vi "GetAllPropertyName.vi"(11 "JSON":string) -> (3 "output array":string[](array[string]))   [LabVIEW 2017]
uses:
  <vilib>/JDP Science/JSONtext/JSONtext.lvlib
  69925c48-c7bb-4434-a24c-5319c87c29c6.vi
  955f1e7d-53c6-494f-b1ae-88a05e9839de.vi
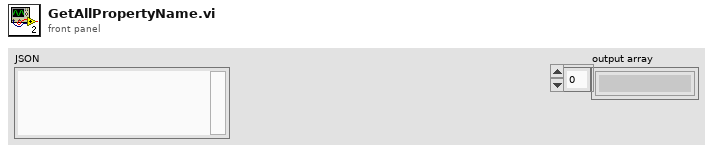
[diagram p1: front panel]
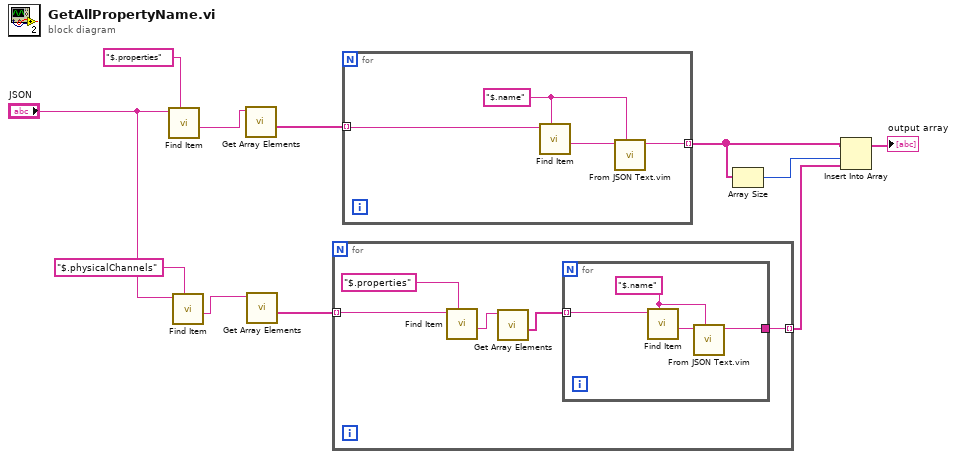
[diagram p0: block diagram]
diagram:
  n1 = call <vilib>:"Find Item.vi"("$Path or Item Name"="$.properties", "JSON"="JSON") -> ("<JSON>"=w10:string)  [unwired: 6 in, 3 out]
  n2 = call <vilib>:"Find Item.vi"("$Path or Item Name"="$.physicalChannels", "JSON"="JSON") -> ("<JSON>"=w6:string)  [unwired: 6 in, 3 out]
  n3 = call <vilib>:"Get Array Elements.vi"("JSON"=w10) -> ("<JSON>"=w9:string[])  [unwired: 8 in, 2 out]
  n4 = call <vilib>:"Get Array Elements.vi"("JSON"=w6) -> ("<JSON>"=w5:string[])  [unwired: 8 in, 2 out]
  n5 = for {
    tunnel: w5 -> [w16] mode=indexing
    tunnel: [w14] -> w2 mode=indexing
    n6 = call <vilib>:"Find Item.vi"("$Path or Item Name"="$.properties", "JSON"=w16) -> ("<JSON>"=w13:string)  [unwired: 6 in, 3 out]
    n7 = call <vilib>:"Get Array Elements.vi"("JSON"=w13) -> ("<JSON>"=w12:string[])  [unwired: 8 in, 2 out]
    n8 = for {
      tunnel: [w18] -> w14
      tunnel: w12 -> [w19] mode=indexing
      w17 = "$.name" ("$Path or Item Name")
      n9 = call <vilib>:"Find Item.vi"("$Path or Item Name"=w17, "JSON"=w19) -> ("<JSON>"=w20:string)  [unwired: 6 in, 3 out]
      n10 = call "From JSON Text.vim"("Data Type and Default Value"=w17, "JSON"=w20) -> ("Data out"=w18:string)  [unwired: 8 in, 1 out]
    }
  }
  n11 = for {
    tunnel: w9 -> [w24] mode=indexing
    tunnel: [w22] -> w4 mode=indexing
    w21 = "$.name" ("$Path or Item Name")
    n12 = call <vilib>:"Find Item.vi"("$Path or Item Name"=w21, "JSON"=w24) -> ("<JSON>"=w23:string)  [unwired: 6 in, 3 out]
    n13 = call "From JSON Text.vim"("Data Type and Default Value"=w21, "JSON"=w23) -> ("Data out"=w22:string)  [unwired: 8 in, 1 out]
  }
  n14 = Array Size(array=w4) -> (size(s)=w3:i32)
  n15 = Insert Into Array(array=w4, index=w3, new element=w2) -> (→"output array":string[])
